vi "write_metadata_atributes.vi"(5 "Group ID":string, 6 "error in (no error)":errorcluster, 8 "Cluster":T1 {"File Location" items=["Unknown"=-5, "IDL Processing"=-4, "Writing from Queue"=-3, "Labview Files"=-2, "Retry Labview files"=-1, "Local Cache "=0, "Old Storage"=1, "Storage"=2]; "Estimate Source" items=["Any Source."=-2, "No Shot"=-1, "Basic Labview Estimate"=0, "IDL Estimate From Andrew"=1, "IDL Estimate From Tobin"=2, "Old Metadata"=3]}, 9 "group ref":i32) -> (0 "error out":errorcluster, 3 "group ref out":i32)   [LabVIEW 2013]
uses:
  Public API/Query_Dust_Event.ctl
  Estimate_source.ctl
  File_location.ctl
  <vilib>/addons/h5labview/H5Attrib.lvlib
panel:
  # "Dust Event"
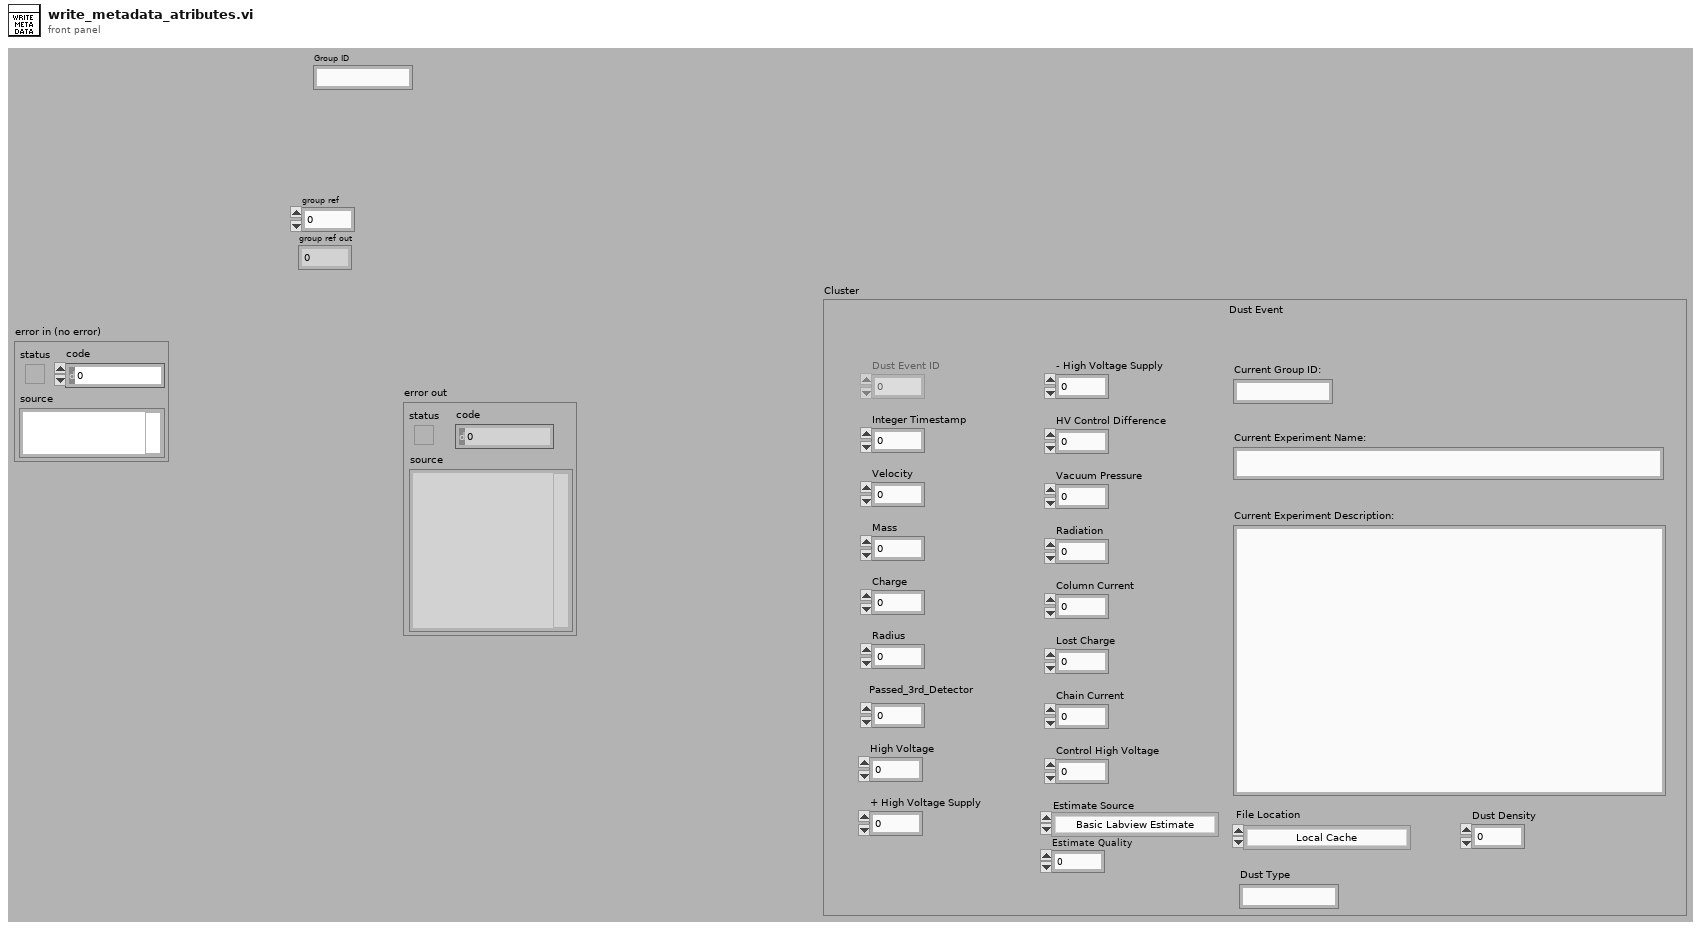
[diagram p1: front panel]
types:
  T1 = typedef "Query_Dust_Event.ctl" = cluster{"Dust Event ID":i64, "Integer Timestamp":i64, "Velocity":sgl, "Mass":sgl, "Charge":sgl, "Radius":sgl, "Passed_3rd_Detector":i8, "High Voltage":sgl, "+ High Voltage Supply":sgl, "- High Voltage Supply":sgl, "HV Control Difference":sgl, "Vacuum Pressure":sgl, "Radiation":sgl, "Column Current":sgl, "Lost Charge":sgl, "Chain Current":sgl, "Control High Voltage":sgl, "Current Group ID:":string, "Current Experiment Name:":string, "Current Experiment Description:":string, "Estimate Source":T2, "Estimate Quality":sgl, "File Location":T3, "Dust Type":string, "Dust Density":sgl}
  T2 = typedef "Estimate_source.ctl" = i8
  T3 = typedef "File_location.ctl" = i8
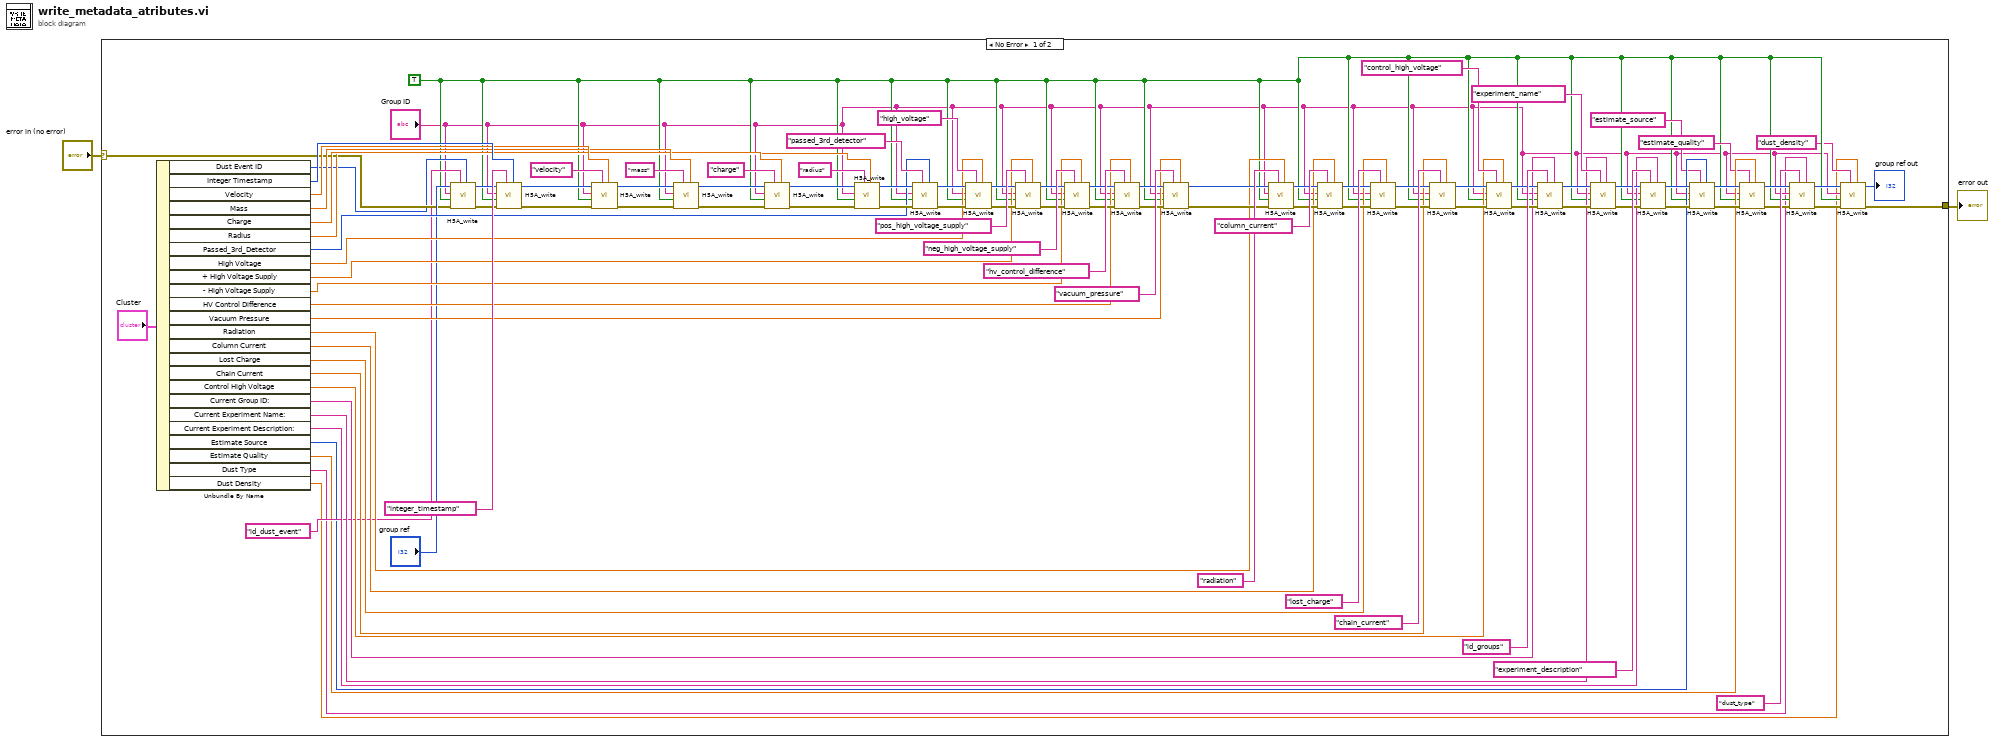
[diagram p0: block diagram]
diagram:
  n1 = case shown="No Error" "error in (no error)" {
    selector: "error in (no error)" -> [w25 w104]
    tunnel: [w9 w104] -> w1
    frame No Error {
      w7 = TRUE
      n2 = Unbundle By Name("Cluster") -> ("Dust Event ID"=w24:i64, "Integer Timestamp"=w102:i64, "Velocity"=w100:sgl, "Mass"=w94:sgl, "Charge"=w45:sgl, "Radius"=w44:sgl, "Passed_3rd_Detector"=w42:i8, "High Voltage"=w41:sgl, "+ High Voltage Supply"=w40:sgl, "- High Voltage Supply"=w39:sgl, "HV Control Difference"=w38:sgl, "Vacuum Pressure"=w37:sgl, "Radiation"=w36:sgl, "Column Current"=w35:sgl, "Lost Charge"=w34:sgl, "Chain Current"=w33:sgl, "Control High Voltage"=w32:sgl, "Current Group ID:"=w31:string, "Current Experiment Name:"=w30:string, "Current Experiment Description:"=w29:string, "Estimate Source"=w18:T2, "Estimate Quality"=w17:sgl, "Dust Type"=w5:string, "Dust Density"=w3:sgl)
      n3 = call <vilib>:"H5A_write.vi"("value"=w24, "attrib_name"="id_dust_event", "error in (no error)"=w25, "overwrite? (F)"=w7, "obj_name"="Group ID", "ref"="group ref") -> ("error out"=w26:errorcluster, "ref out"=w28:i32)  [unwired: 2 in]
      n4 = call <vilib>:"H5A_write.vi"("value"=w102, "attrib_name"="integer_timestamp", "error in (no error)"=w26, "overwrite? (F)"=w7, "obj_name"="Group ID", "ref"=w28) -> ("error out"=w98:errorcluster, "ref out"=w99:i32)  [unwired: 2 in]
      n5 = call <vilib>:"H5A_write.vi"("value"=w100, "attrib_name"="velocity", "error in (no error)"=w98, "overwrite? (F)"=w7, "obj_name"="Group ID", "ref"=w99) -> ("error out"=w96:errorcluster, "ref out"=w97:i32)  [unwired: 2 in]
      n6 = call <vilib>:"H5A_write.vi"("value"=w94, "attrib_name"="mass", "error in (no error)"=w96, "overwrite? (F)"=w7, "obj_name"="Group ID", "ref"=w97) -> ("error out"=w77:errorcluster, "ref out"=w93:i32)  [unwired: 2 in]
      n7 = call <vilib>:"H5A_write.vi"("value"=w45, "attrib_name"="charge", "error in (no error)"=w77, "overwrite? (F)"=w7, "obj_name"="Group ID", "ref"=w93) -> ("error out"=w76:errorcluster, "ref out"=w60:i32)  [unwired: 2 in]
      n8 = call <vilib>:"H5A_write.vi"("value"=w44, "attrib_name"="radius", "error in (no error)"=w76, "overwrite? (F)"=w7, "obj_name"="Group ID", "ref"=w60) -> ("error out"=w43:errorcluster, "ref out"=w59:i32)  [unwired: 2 in]
      n9 = call <vilib>:"H5A_write.vi"("value"=w42, "attrib_name"="passed_3rd_detector", "error in (no error)"=w43, "overwrite? (F)"=w7, "obj_name"="Group ID", "ref"=w59) -> ("error out"=w75:errorcluster, "ref out"=w58:i32)  [unwired: 2 in]
      n10 = call <vilib>:"H5A_write.vi"("value"=w41, "attrib_name"="high_voltage", "error in (no error)"=w75, "overwrite? (F)"=w7, "obj_name"="Group ID", "ref"=w58) -> ("error out"=w74:errorcluster, "ref out"=w57:i32)  [unwired: 2 in]
      n11 = call <vilib>:"H5A_write.vi"("value"=w40, "attrib_name"="pos_high_voltage_supply", "error in (no error)"=w74, "overwrite? (F)"=w7, "obj_name"="Group ID", "ref"=w57) -> ("error out"=w73:errorcluster, "ref out"=w56:i32)  [unwired: 2 in]
      n12 = call <vilib>:"H5A_write.vi"("value"=w39, "attrib_name"="neg_high_voltage_supply", "error in (no error)"=w73, "overwrite? (F)"=w7, "obj_name"="Group ID", "ref"=w56) -> ("error out"=w72:errorcluster, "ref out"=w55:i32)  [unwired: 2 in]
      n13 = call <vilib>:"H5A_write.vi"("value"=w38, "attrib_name"="hv_control_difference", "error in (no error)"=w72, "overwrite? (F)"=w7, "obj_name"="Group ID", "ref"=w55) -> ("error out"=w71:errorcluster, "ref out"=w54:i32)  [unwired: 2 in]
      n14 = call <vilib>:"H5A_write.vi"("value"=w37, "attrib_name"="vacuum_pressure", "error in (no error)"=w71, "overwrite? (F)"=w7, "obj_name"="Group ID", "ref"=w54) -> ("error out"=w70:errorcluster, "ref out"=w53:i32)  [unwired: 2 in]
      n15 = call <vilib>:"H5A_write.vi"("value"=w36, "attrib_name"="radiation", "error in (no error)"=w70, "overwrite? (F)"=w7, "obj_name"="Group ID", "ref"=w53) -> ("error out"=w69:errorcluster, "ref out"=w52:i32)  [unwired: 2 in]
      n16 = call <vilib>:"H5A_write.vi"("value"=w35, "attrib_name"="column_current", "error in (no error)"=w69, "overwrite? (F)"=w7, "obj_name"="Group ID", "ref"=w52) -> ("error out"=w68:errorcluster, "ref out"=w51:i32)  [unwired: 2 in]
      n17 = call <vilib>:"H5A_write.vi"("value"=w34, "attrib_name"="lost_charge", "error in (no error)"=w68, "overwrite? (F)"=w7, "obj_name"="Group ID", "ref"=w51) -> ("error out"=w67:errorcluster, "ref out"=w50:i32)  [unwired: 2 in]
      n18 = call <vilib>:"H5A_write.vi"("value"=w33, "attrib_name"="chain_current", "error in (no error)"=w67, "overwrite? (F)"=w7, "obj_name"="Group ID", "ref"=w50) -> ("error out"=w66:errorcluster, "ref out"=w49:i32)  [unwired: 2 in]
      n19 = call <vilib>:"H5A_write.vi"("value"=w32, "attrib_name"="control_high_voltage", "error in (no error)"=w66, "overwrite? (F)"=w7, "obj_name"="Group ID", "ref"=w49) -> ("error out"=w65:errorcluster, "ref out"=w48:i32)  [unwired: 2 in]
      n20 = call <vilib>:"H5A_write.vi"("value"=w31, "attrib_name"="id_groups", "error in (no error)"=w65, "overwrite? (F)"=w7, "obj_name"="Group ID", "ref"=w48) -> ("error out"=w64:errorcluster, "ref out"=w47:i32)  [unwired: 2 in]
      n21 = call <vilib>:"H5A_write.vi"("value"=w30, "attrib_name"="experiment_name", "error in (no error)"=w64, "overwrite? (F)"=w7, "obj_name"="Group ID", "ref"=w47) -> ("error out"=w62:errorcluster, "ref out"=w46:i32)  [unwired: 2 in]
      n22 = call <vilib>:"H5A_write.vi"("value"=w29, "attrib_name"="experiment_description", "error in (no error)"=w62, "overwrite? (F)"=w7, "obj_name"="Group ID", "ref"=w46) -> ("error out"=w19:errorcluster, "ref out"=w20:i32)  [unwired: 2 in]
      n23 = call <vilib>:"H5A_write.vi"("value"=w18, "attrib_name"="estimate_source", "error in (no error)"=w19, "overwrite? (F)"=w7, "obj_name"="Group ID", "ref"=w20) -> ("error out"=w21:errorcluster, "ref out"=w22:i32)  [unwired: 2 in]
      n24 = call <vilib>:"H5A_write.vi"("value"=w17, "attrib_name"="estimate_quality", "error in (no error)"=w21, "overwrite? (F)"=w7, "obj_name"="Group ID", "ref"=w22) -> ("error out"=w8:errorcluster, "ref out"=w14:i32)  [unwired: 2 in]
      n25 = call <vilib>:"H5A_write.vi"("value"=w5, "attrib_name"="dust_type", "error in (no error)"=w8, "overwrite? (F)"=w7, "obj_name"="Group ID", "ref"=w14) -> ("error out"=w10:errorcluster, "ref out"=w13:i32)  [unwired: 2 in]
      n26 = call <vilib>:"H5A_write.vi"("value"=w3, "attrib_name"="dust_density", "error in (no error)"=w10, "overwrite? (F)"=w7, "obj_name"="Group ID", "ref"=w13) -> ("error out"=w9:errorcluster, "ref out"=→"group ref out":i32)  [unwired: 2 in]
    }
    frame Error {
    }
  }
  "error out" <- w1
